vi "[SubVI]Torque_Measured.vi"(4 "Left Alpha":dbl, 5 "Right Alpha":dbl, 6 "Left Deflection":dbl format="%#_13g", 7 "Right Deflection":dbl format="%#_13g") -> (0 "Left Torque Measured":dbl, 1 "Right Torque Measured":dbl)   [LabVIEW 2017]
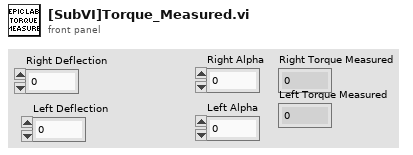
[diagram p1: front panel]
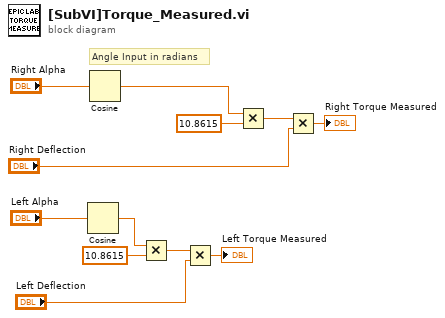
[diagram p0: block diagram]
diagram:
  # "Angle Input in radians"
  n1 = Cosine(x="Left Alpha") -> (cos(x)=w8:dbl)
  n2 = Cosine(x="Right Alpha") -> (cos(x)=w12:dbl)
  n3 = Multiply(x=w8, y=10.8615 ("Right Torque Measured 2")) -> (x*y=w5:dbl)
  n4 = Multiply(x=w5, y="Left Deflection") -> (x*y=→"Left Torque Measured":dbl)
  n5 = Multiply(x=w12, y=10.8615 ("Right Torque Measured 2")) -> (x*y=w9:dbl)
  n6 = Multiply(x=w9, y="Right Deflection") -> (x*y=→"Right Torque Measured":dbl)
